vi "ClearQueue.vi"(0 "Program Interface in":refnum<class "Program Interface.lvclass">, 5 "error in (no error)":errorcluster) -> (14 "Program Interface out":refnum<class "Program Interface.lvclass">, 19 "error out":errorcluster)   [LabVIEW 2016, in "Program Interface.lvclass"]
uses:
  Program Interface.lvclass
  Program Interface.lvclass/Program Interface.ctl
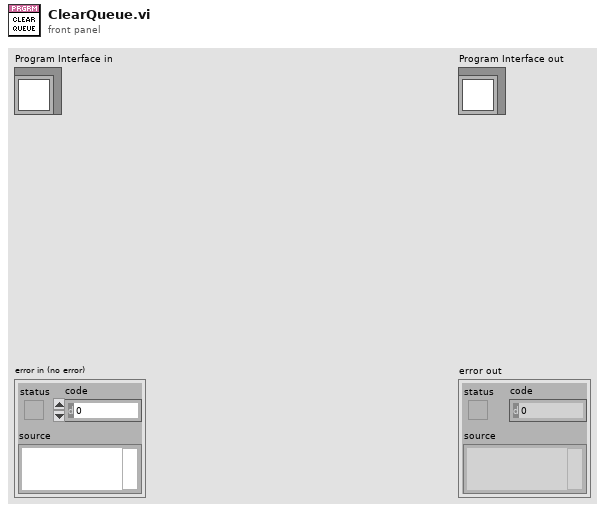
[diagram p1: front panel]
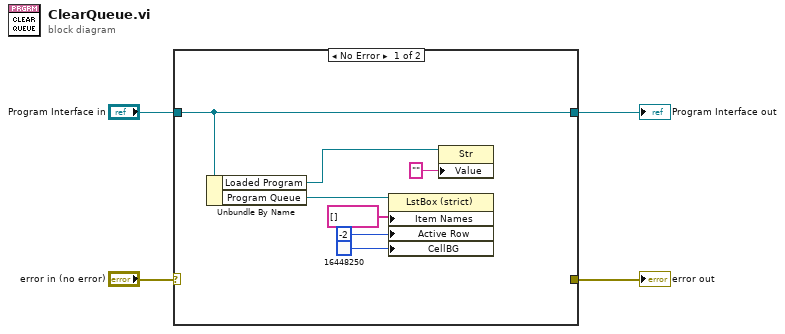
[diagram p0: block diagram]
diagram:
  n1 = case shown="No Error" "error in (no error)" {
    selector: "error in (no error)" -> [_ w13]
    tunnel: [_ w13] -> w3
    tunnel: [w11 w12] -> w1
    tunnel: "Program Interface in" -> [w11 w12]
    frame No Error {
      n2 = Unbundle By Name(w11) -> ("Loaded Program"=w10:refnum<vi>, "Program Queue"=w7:refnum<vi>)
      n3 = property class="LstBox (strict)"(reference=w7, "Item Names"=string[] [], "Active Row"=-2 ("Active Row:Active Row Number"), "CellBG"=u32 16448250) -> ()  [unwired: 1 in, 2 out]
      n4 = property class="Str"(reference=w10, "Value"="") -> ()  [unwired: 1 in, 2 out]
    }
    frame Error {
    }
  }
  "error out" <- w3
  "Program Interface out" <- w1
